vi "OxITC503 _Config_ Set Controller.vi"(2 "Auto Status":T1(ring)=enum."Heater Auto, Gas Manual", 3 "Auto PID (Off)":enum16{"Auto PID Off", "Auto PID On"}(ring), 4 "error in (no error)":errorcluster, 5 "Temperature Control Settings":T2 {"D" format="%.2f"; "I" format="%.2f"; "P" format="%.2f"; "Setpoint" format="%.2f"}, 6 "Sweep Status (Off)":enum16{"Sweep Off", "Sweep On"}(ring), 7 "VISA session":refnum<visa-resource-name>) -> (0 "error out":errorcluster, 1 "VISA session":refnum<visa-resource-name>)   [LabVIEW 2013]
doc: "Allows the user to configurate the ITC503."
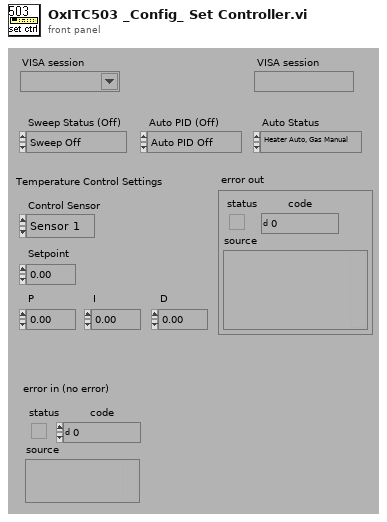
[diagram p1: front panel]
types:
  T1 = enum16{"Heater and gas Manual", "Heater Auto, Gas Manual", "Heater Manual, Gas Auto", "Heater and Gas Auto"}
  T2 = cluster{"Setpoint":dbl, "Control Sensor":enum16{"Sensor 1", "Sensor 2", "Sensor 3"}, "P":dbl, "I":dbl, "D":dbl}
  T3 = enum16{"Local and locked", "Remote and Locked", "Local and unlocked", "Remote and Unlocked"}
  T4 = cluster{"System Status":i32, "Auto Status":enum16{"Heater and gas Manual", "Heater Auto, Gas Manual", "Heater Manual, Gas Auto", "Heater and Gas Auto"}, "Control Status":enum16{"Local and locked", "Remote and Locked", "Local and unlocked", "Remote and Unlocked"}, "Sweep Stage":i32, "Control Sensor":enum16{"Sensor 1", "Sensor 2", "Sensor 3"}, "Auto PID Status":enum16{"Auto PID Off", "Auto PID On"}}
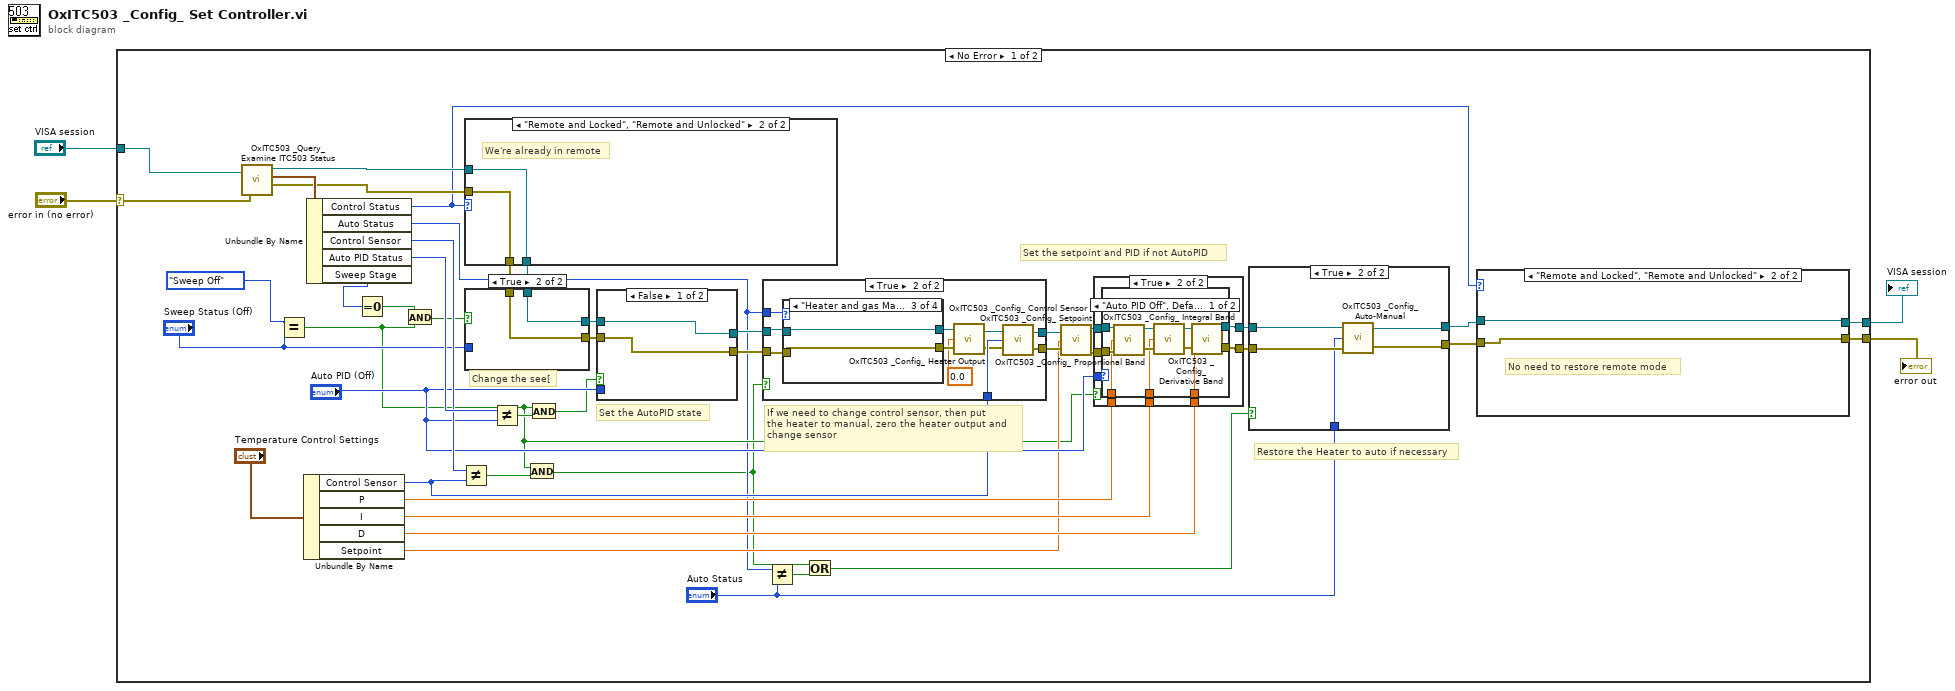
[diagram p0: block diagram]
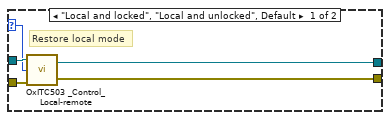
[diagram p4: hidden frame]
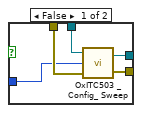
[diagram p5: hidden frame]
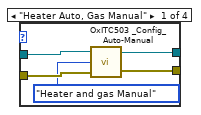
[diagram p8: hidden frame]
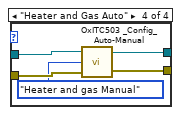
[diagram p10: hidden frame]
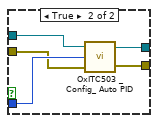
[diagram p11: hidden frame]
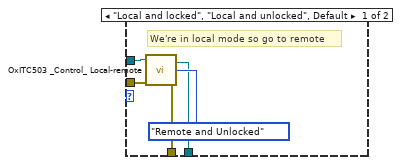
[diagram p12: hidden frame]
diagram:
  n1 = case shown="No Error" "error in (no error)" {
    selector: "error in (no error)" -> [w5 w135]
    tunnel: "VISA session" -> [w29 w136]
    tunnel: [w21 w136] -> w3
    tunnel: [w20 w135] -> w2
    frame No Error {
      # "Restore the Heater to auto if necessary"
      # "Set the setpoint and PID if not AutoPID"
      # "If we need to change control sensor, then put\nthe heater to manual, zero the heater output and\nchange sensor"
      # "Set the AutoPID state"
      # "Change the see["
      n2 = call "OxITC503 _Query_ Examine ITC503 Status.vi"("VISA session"=w29, "error in"=w5) -> ("VISA session"=w48:refnum<visa-resource-name>, "ITC Status"=w49:T4, "error out (no error)"=w47:errorcluster)  [unwired: 1 out]
      n3 = Equal?(x=enum16{"Sweep Off", "Sweep On"}."Sweep Off" ("Sweep Status"), y="Sweep Status (Off)") -> (x = y?=w11:bool)
      n4 = Unbundle By Name("Temperature Control Settings") -> ("Control Sensor"=w41:enum16{"Sensor 1", "Sensor 2", "Sensor 3"}, "P"=w33:dbl, "I"=w32:dbl, "D"=w31:dbl, "Setpoint"=w30:dbl)
      n5 = Unbundle By Name(w49) -> ("Control Status"=w22:T3, "Auto Status"=w9:T1, "Control Sensor"=w44:enum16{"Sensor 1", "Sensor 2", "Sensor 3"}, "Auto PID Status"=w46:enum16{"Auto PID Off", "Auto PID On"}, "Sweep Stage"=w16:i32)
      n6 = Equal To 0?(x=w16) -> (x = 0?=w17:bool)
      n7 = And(x=w17, y=w11) -> (x .and. y?=w15:bool)
      n8 = Not Equal?(x=w44, y=w41) -> (x != y?=w12:bool)
      n9 = case shown="\"Remote and Locked\", \"Remote and Unlocked\"" w22 {
        tunnel: w48 -> [w132 w134]
        tunnel: w47 -> [w131 w133]
        tunnel: [w129 w134] -> w26
        tunnel: [w128 w133] -> w25
        frame "Local and locked", "Local and unlocked", Default {
          # "We're in local mode so go to remote"
          n10 = call "OxITC503 _Control_ Local-remote.vi"("error in"=w131, "Control Status"=T3."Remote and Unlocked", "VISA session"=w132) -> ("error out (no error)"=w128:errorcluster, "VISA session"=w129:refnum<visa-resource-name>)
        }
        frame "Remote and Locked", "Remote and Unlocked" {
          # "We're already in remote"
        }
      }
      n11 = case shown="True" w15 {
        tunnel: [w84 w86] -> w28
        tunnel: [w83 w85] -> w27
        tunnel: w26 -> [w82 w86]
        tunnel: w25 -> [w81 w85]
        tunnel: "Sweep Status (Off)" -> [w80 _]
        frame False {
          n12 = call "OxITC503 _Config_ Sweep.vi"("error in"=w81, "Sweep Status"=w80, "VISA session"=w82) -> ("error out (no error)"=w83:errorcluster, "VISA session"=w84:refnum<visa-resource-name>)
        }
        frame True {
        }
      }
      n13 = Not Equal?(x=w46, y="Auto PID (Off)") -> (x != y?=w14:bool)
      n14 = And(x=w11, y=w12) -> (x .and. y?=w7:bool)
      n15 = And(x=w11, y=w14) -> (x .and. y?=w13:bool)
      n16 = case shown="False" w13 {
        tunnel: "Auto PID (Off)" -> [_ w127]
        tunnel: [w122 w126] -> w43
        tunnel: [w121 w125] -> w42
        tunnel: w28 -> [w122 w124]
        tunnel: w27 -> [w121 w123]
        frame False {
        }
        frame True {
          n17 = call "OxITC503 _Config_ Auto PID.vi"("error in"=w123, "Auto PID Status"=w127, "VISA session"=w124) -> ("error out (no error)"=w125:errorcluster, "VISA session"=w126:refnum<visa-resource-name>)
        }
      }
      n18 = case shown="True" w7 {
        tunnel: w43 -> [w95 w106]
        tunnel: w42 -> [w94 w105]
        tunnel: w9 -> [_ w103]
        tunnel: w41 -> [_ w104]
        tunnel: [w95 w97] -> w39
        tunnel: [w94 w96] -> w38
        frame False {
        }
        frame True {
          n19 = case shown="\"Heater and gas Manual\"" w103 {
            tunnel: w106 -> [w111 w113 w115 w120]
            tunnel: w105 -> [w110 w112 w114 w119]
            tunnel: [w108 w112 w114 w117] -> w100
            tunnel: [w107 w113 w115 w116] -> w102
            frame "Heater Auto, Gas Manual" {
              n20 = call "OxITC503 _Config_ Auto-Manual.vi"("error in"=w110, "Auto Status"=T1."Heater and gas Manual", "VISA session"=w111) -> ("error out (no error)"=w108:errorcluster, "VISA session"=w107:refnum<visa-resource-name>)
            }
            frame "Heater Manual, Gas Auto" {
            }
            frame "Heater and gas Manual" {
            }
            frame "Heater and Gas Auto" {
              n21 = call "OxITC503 _Config_ Auto-Manual.vi"("error in"=w119, "Auto Status"=T1."Heater and gas Manual", "VISA session"=w120) -> ("error out (no error)"=w117:errorcluster, "VISA session"=w116:refnum<visa-resource-name>)
            }
          }
          n22 = call "OxITC503 _Config_ Heater Output.vi"("error in"=w100, "Heater Output (%)"=0.0, "VISA session"=w102) -> ("error out (no error)"=w99:errorcluster, "VISA session"=w101:refnum<visa-resource-name>)
          n23 = call "OxITC503 _Config_ Control Sensor.vi"("error in"=w99, "Control Sensor"=w104, "VISA session"=w101) -> ("error out (no error)"=w96:errorcluster, "VISA session"=w97:refnum<visa-resource-name>)
        }
      }
      n24 = Not Equal?(x=w9, y="Auto Status") -> (x != y?=w8:bool)
      n25 = Or(x=w7, y=w8) -> (x .or. y?=w6:bool)
      n26 = call "OxITC503 _Config_ Setpoint.vi"("error in"=w38, "Setpoint"=w30, "VISA session"=w39) -> ("error out (no error)"=w36:errorcluster, "VISA session"=w37:refnum<visa-resource-name>)
      n27 = case shown="True" w11 {
        tunnel: "Auto PID (Off)" -> [_ w59]
        tunnel: w37 -> [w51 w58]
        tunnel: w36 -> [w50 w57]
        tunnel: [w51 w56] -> w35
        tunnel: [w50 w55] -> w34
        tunnel: w33 -> [_ w54]
        tunnel: w32 -> [_ w53]
        tunnel: w31 -> [_ w52]
        frame False {
        }
        frame True {
          n28 = case shown="\"Auto PID Off\", Default" w59 {
            tunnel: w58 -> [w70 w72]
            tunnel: w57 -> [w69 w71]
            tunnel: [w64 w72] -> w56
            tunnel: [w63 w71] -> w55
            tunnel: w54 -> [w62 _]
            tunnel: w53 -> [w61 _]
            tunnel: w52 -> [w60 _]
            frame "Auto PID Off", Default {
              n29 = call "OxITC503 _Config_ Proportional Band.vi"("error in"=w69, "Proportional Band Value"=w62, "VISA session"=w70) -> ("error out (no error)"=w67:errorcluster, "VISA session"=w68:refnum<visa-resource-name>)
              n30 = call "OxITC503 _Config_ Integral Band.vi"("error in"=w67, "Integral Band Value"=w61, "VISA session"=w68) -> ("error out (no error)"=w65:errorcluster, "VISA session"=w66:refnum<visa-resource-name>)
              n31 = call "OxITC503 _Config_ Derivative Band.vi"("error in"=w65, "Derivative Band Value"=w60, "VISA session"=w66) -> ("error out (no error)"=w63:errorcluster, "VISA session"=w64:refnum<visa-resource-name>)
            }
            frame "Auto PID On" {
            }
          }
        }
      }
      n32 = case shown="True" w6 {
        tunnel: w35 -> [w88 w93]
        tunnel: w34 -> [w87 w92]
        tunnel: [w87 w90] -> w23
        tunnel: [w88 w91] -> w24
        tunnel: "Auto Status" -> [_ w89]
        frame False {
        }
        frame True {
          n33 = call "OxITC503 _Config_ Auto-Manual.vi"("error in"=w92, "Auto Status"=w89, "VISA session"=w93) -> ("error out (no error)"=w90:errorcluster, "VISA session"=w91:refnum<visa-resource-name>)
        }
      }
      n34 = case shown="\"Remote and Locked\", \"Remote and Unlocked\"" w22 {
        selector: w22 -> [w75 _]
        tunnel: w24 -> [w77 w79]
        tunnel: w23 -> [w76 w78]
        tunnel: [w74 w79] -> w21
        tunnel: [w73 w78] -> w20
        frame "Local and locked", "Local and unlocked", Default {
          # "Restore local mode"
          n35 = call "OxITC503 _Control_ Local-remote.vi"("error in"=w76, "Control Status"=w75, "VISA session"=w77) -> ("error out (no error)"=w73:errorcluster, "VISA session"=w74:refnum<visa-resource-name>)
        }
        frame "Remote and Locked", "Remote and Unlocked" {
          # "No need to restore remote mode"
        }
      }
    }
    frame Error {
    }
  }
  "error out" <- w2
  "VISA session" <- w3
